vi "V_GetShapeResultNames.vi"(10 "SetParameter":T1={"Enum_ShapeType"=enum."Circles", "MaxParticle"=1, "Descriptor"={"Set 1"=100.0, "Set 2"=10.0, "Set 3"=200.0, "Set 4"=10.0}, "Match Options"={"Rotation"=TRUE, "Scale"=FALSE, "Occlusion"=FALSE, "Range Settings"=[{"Match Constraints"=0, "Min"=0.0, "Max"=360.0}]}, "Curve Parameters"={"Extraction Mode"=0, "Edge Threshold"=75, "Edge Filter Size"=1, "Min Length"=25, "Row Search Step Size"=15, "Col Search Step Size"=15, "Max Endpoint Gap"=10, "Closed"=FALSE, "Subpixel"=FALSE}, " score"=500.0} {"score" format="%#_15g"; "Curve Parameters"."Extraction Mode" items=["Normal", "Uniform Regions"]; "Curve Parameters"."Edge Filter Size" items=["Fine", "Normal"]; "Match Options"."Range Settings"."Match Constraints" items=["Rotation Angle (degrees)", "Scale Factor (%)", "Occlusion (%)"]}, 11 "ROI_Name":string="ROI1") -> (3 "ResultNames":string[](array[string]))   [LabVIEW 2019]
uses:
  Controls/Circle/Analysis_Circle_Result.ctl
  Controls/ShapeDectect/Analysis_ShapeDectect_Parameter.ctl
panel:
  in  "Tab Control":T2(tab)
  in  "Circles":T3
  in  "Ellipses":T4
  in  "Lines":T5
  in  "Rectangles":T6
  in  "Analysis_Clamp_Result":T7 {"Fitted Circle"."Average SNR (dB)" format="%.2f"; "Fitted Circle"."Average Strength" format="%.2f"; "Fitted Circle"."Roundness (Real-World)" format="%.2f"; "Fitted Circle"."Radius (Real-World)" format="%.2f"; "Fitted Circle"."Center (Real-World)"."Y" format="%.2f"; "Fitted Circle"."Center (Real-World)"."X" format="%.2f"; "Fitted Circle"."Radius (Pixels)" format="%.2f"; "Fitted Circle"."Center (Pixels)"."Y" format="%.2f"; "Fitted Circle"."Center (Pixels)"."X" format="%.2f"}
  out "error out":errorcluster
  in  "error in (no error)":errorcluster
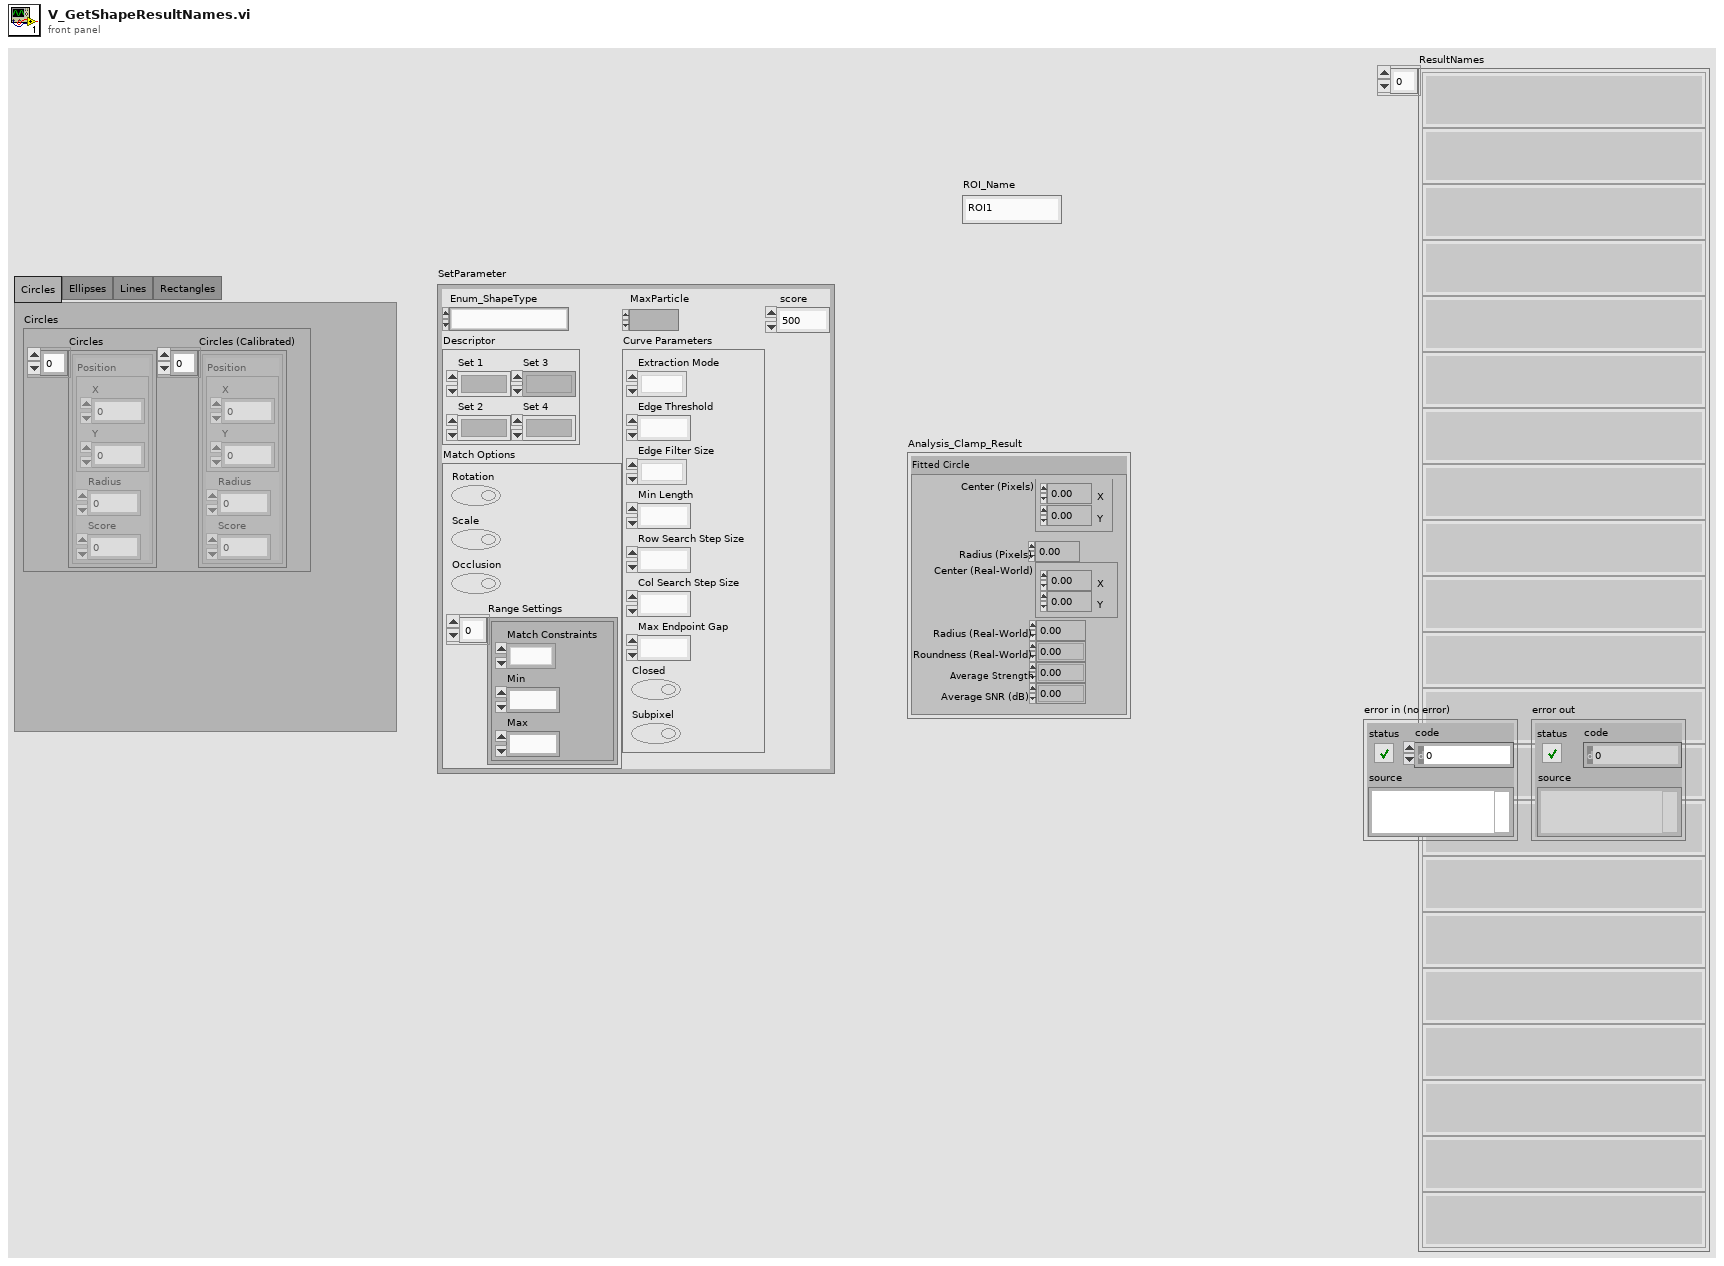
[diagram p1: front panel]
types:
  T1 = typedef "Analysis_ShapeDectect_Parameter.ctl" = cluster{"Enum_ShapeType":enum16{"Circles", "Ellipses", "Lines", "Rectangles"}, "MaxParticle":i32, "Descriptor":cluster{"Set 1":dbl, "Set 2":dbl, "Set 3":dbl, "Set 4":dbl}, "Match Options":cluster{"Rotation":bool, "Scale":bool, "Occlusion":bool, "Range Settings":cluster{"Match Constraints":u32, "Min":dbl, "Max":dbl}[]}, "Curve Parameters":cluster{"Extraction Mode":u32, "Edge Threshold":i32, "Edge Filter Size":u32, "Min Length":i32, "Row Search Step Size":i32, "Col Search Step Size":i32, "Max Endpoint Gap":i32, "Closed":bool, "Subpixel":bool}, " score":dbl}
  T2 = enum32{"Circles", "Ellipses", "Lines", "Rectangles"}
  T3 = cluster{"Circles":cluster{"Position":cluster{"X":sgl, "Y":sgl}, "Radius":dbl, "Score":dbl}[], "Circles (Calibrated)":cluster{"Position":cluster{"X":sgl, "Y":sgl}, "Radius":dbl, "Score":dbl}[]}
  T4 = cluster{"Pixel":cluster{"Position":cluster{"X":sgl, "Y":sgl}, "Angle":dbl, "Major Radius":dbl, "Minor Radius":dbl, "Score":dbl}[], "Ellipses (Calibrated)":cluster{"Position":cluster{"X":sgl, "Y":sgl}, "Orientation":dbl, "Major Radius":dbl, "Minor Radius":dbl, "Score":dbl}[]}
  T5 = cluster{"Lines":cluster{"Start Point":cluster{"X":sgl, "Y":sgl}, "End Point":cluster{"X":sgl, "Y":sgl}, "Length":dbl, "Angle":dbl, "Score":dbl}[], "Lines Calibrated":cluster{"Start Point":cluster{"X":sgl, "Y":sgl}, "End Point":cluster{"X":sgl, "Y":sgl}, "Length":dbl, "Orientation":dbl, "Score":dbl}[]}
  T6 = cluster{"Rectangles":cluster{"Corners":cluster{"X":sgl, "Y":sgl}[], "Angle":dbl, "Width":dbl, "Height":dbl, "Score":dbl}[], "Rectangles Calibrated":cluster{"Corners":cluster{"X":sgl, "Y":sgl}[], "Angle":dbl, "Width":dbl, "Height":dbl, "Score":dbl}[]}
  T7 = typedef "Analysis_Circle_Result.ctl" = cluster{"Fitted Circle":cluster{"Center (Pixels)":cluster{"X":sgl, "Y":sgl}, "Radius (Pixels)":dbl, "Center (Real-World)":cluster{"X":sgl, "Y":sgl}, "Radius (Real-World)":dbl, "Roundness (Real-World)":dbl, "Average Strength":dbl, "Average SNR (dB)":dbl}}
  T8 = enum16{"Circles", "Ellipses", "Lines", "Rectangles"}
  T9 = cluster{"Position":cluster{"X":sgl, "Y":sgl}, "Angle":dbl, "Major Radius":dbl, "Minor Radius":dbl, "Score":dbl}
  T10 = cluster{"Start Point":cluster{"X":sgl, "Y":sgl}, "End Point":cluster{"X":sgl, "Y":sgl}, "Length":dbl, "Angle":dbl, "Score":dbl}
  T11 = cluster{"Corners":cluster{"X":sgl, "Y":sgl}[], "Angle":dbl, "Width":dbl, "Height":dbl, "Score":dbl}
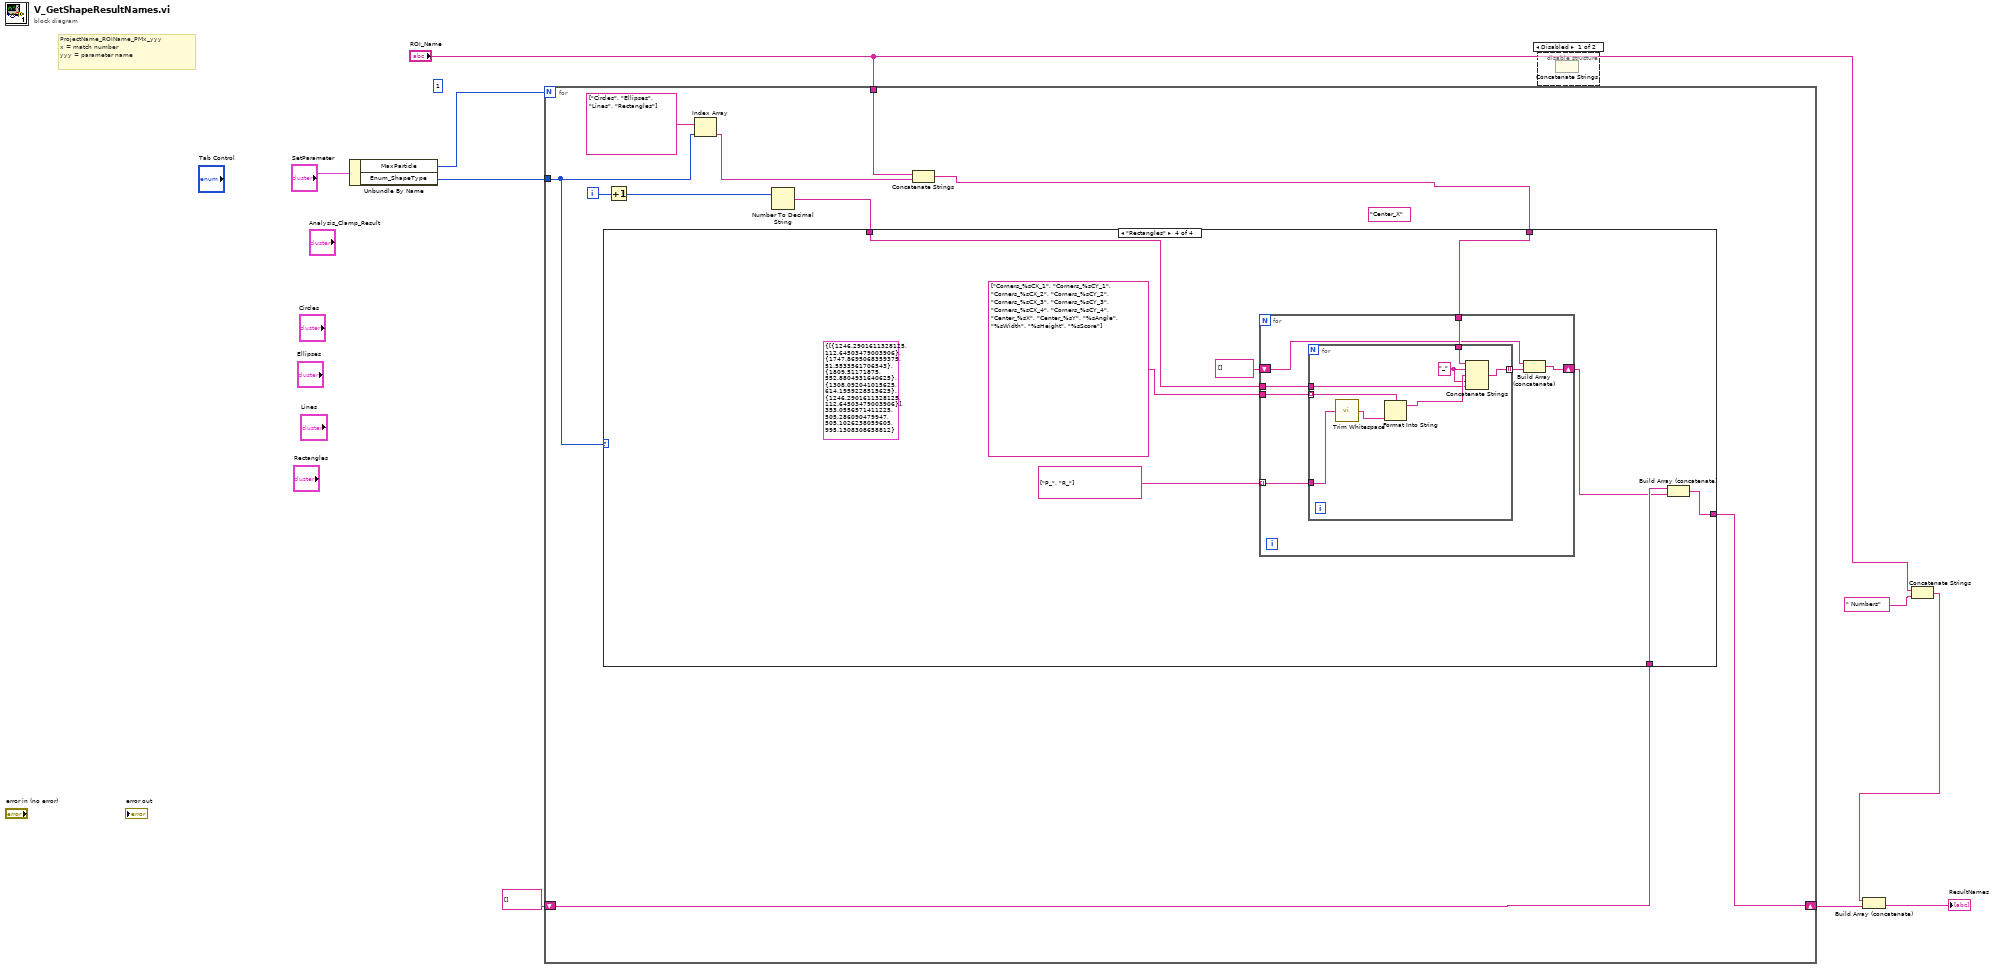
[diagram p0: block diagram]
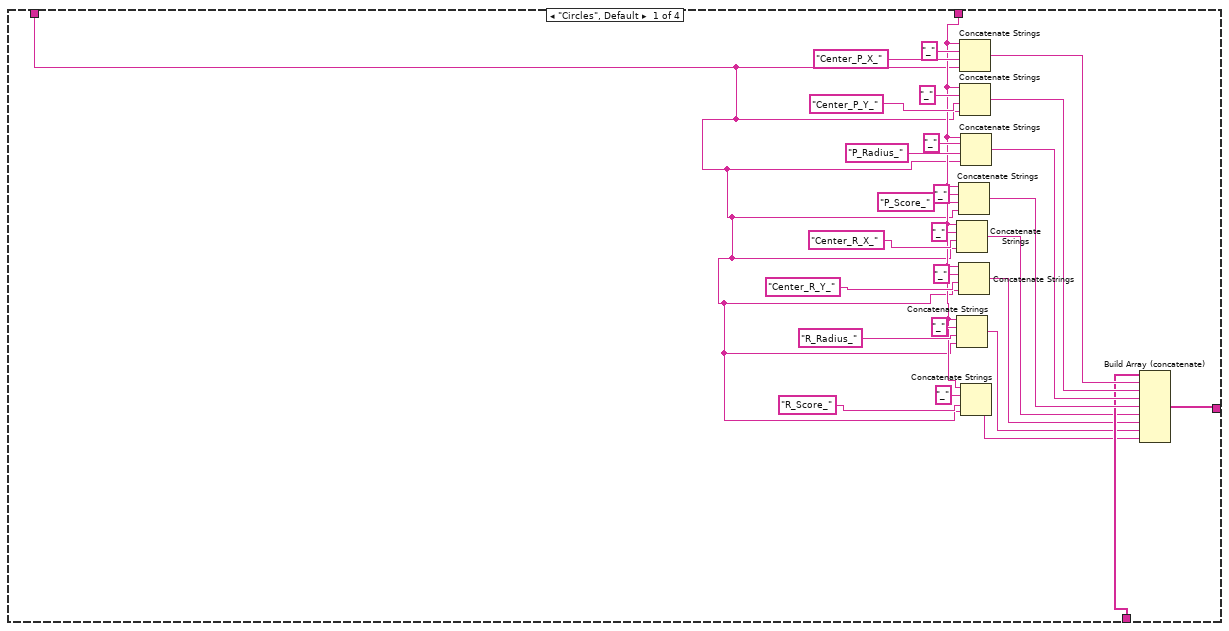
[diagram p3: hidden frame]
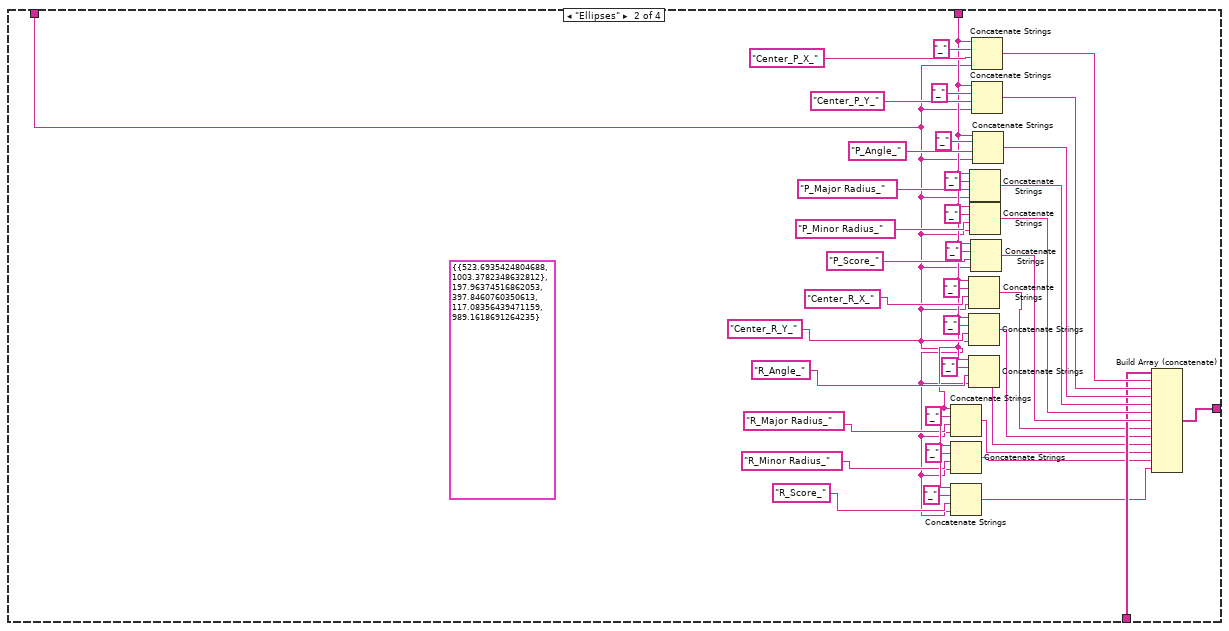
[diagram p4: hidden frame]
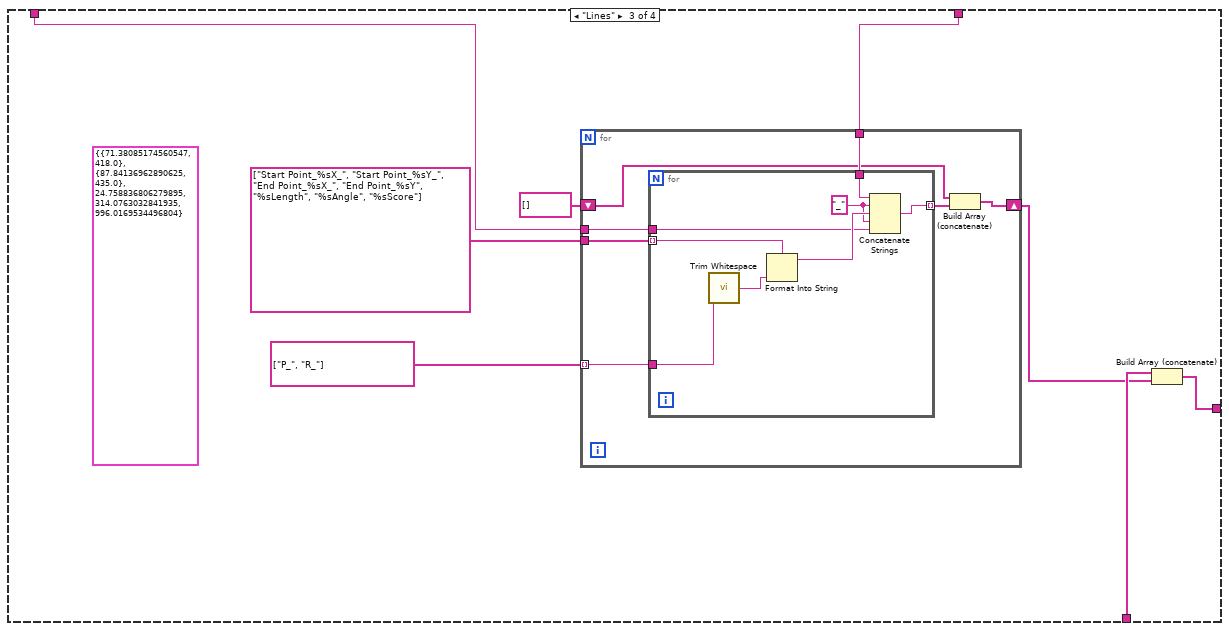
[diagram p5: hidden frame]
diagram:
  (unwired) 1 ("x")
  # "ProjectName_ROIName_PMx_yyy\nx = match number\nyyy = parameter name"
  n1 = Unbundle By Name("SetParameter") -> ("MaxParticle"=w2:i32, "Enum_ShapeType"=w6:T8)
  n2 = for {
    N: w2 -> [_]
    tunnel: "ROI_Name" -> [w18]
    shift-right: [w15] -> w8
    shift-left: string[] [] -> [w16]
    tunnel: w6 -> [w11]
    i -> [w17]
    (unwired) "Center_X" ("string")
    n3 = Increment(x=w17) -> (x+1=w19:i32)
    n4 = Index Array(array=string[] ["Circles", "Ellipses", "Lines", "Rectangles"] ("Array"), index=w11) -> (element=w12:string)
    n5 = Number To Decimal String(number=w19) -> (decimal integer string=w10:string)  [unwired: 1 in]
    n6 = Concatenate Strings(w18, w12) -> (w14:string)
    n7 = case shown="\"Rectangles\"" w11 {
      tunnel: w16 -> [w35 w55 w94 w117]
      tunnel: [w36 w87 w95 w118] -> w15
      tunnel: w14 -> [w26 w60 w91 w115]
      tunnel: w10 -> [w20 w48 w88 w111]
      frame "Circles", Default {
        n8 = Concatenate Strings(w26, "_" ("string"), "Center_R_X_" ("string"), w20) -> (w24:string)
        n9 = Concatenate Strings(w26, "_" ("string"), "R_Radius_" ("string"), w20) -> (w22:string)
        n10 = Concatenate Strings(w26, "_" ("string"), "P_Score_" ("string"), w20) -> (w45:string)
        n11 = Concatenate Strings(w26, "_" ("string"), "Center_R_Y_" ("string"), w20) -> (w23:string)
        n12 = Concatenate Strings(w26, "_" ("string"), "Center_P_X_" ("string"), w20) -> (w47:string)
        n13 = Concatenate Strings(w26, "_" ("string"), "Center_P_Y_" ("string"), w20) -> (w46:string)
        n14 = Concatenate Strings(w26, "_", "P_Radius_" ("string"), w20) -> (w37:string)
        n15 = Concatenate Strings(w26, "_" ("string"), "R_Score_" ("string"), w20) -> (w21:string)
        n16 = Build Array (concatenate)(w35, w47, w46, w37, w45, w24, w23, w22, w21) -> (w36:string[])
      }
      frame "Ellipses" {
        (unwired) T9 {"Position"={"X"=523.69354, "Y"=1003.37823}, "Angle"=197.96374516862053, "Major Radius"=397.8460760350613, "Minor Radius"=117.08356439471159, "Score"=989.1618691264235} ("Circle Descriptor")
        n17 = Concatenate Strings(w60, "_" ("string"), "R_Major Radius_" ("string"), w48) -> (w51:string)
        n18 = Concatenate Strings(w60, "_" ("string"), "R_Minor Radius_" ("string"), w48) -> (w50:string)
        n19 = Concatenate Strings(w60, "_" ("string"), "R_Score_" ("string"), w48) -> (w49:string)
        n20 = Concatenate Strings(w60, "_" ("string"), "Center_R_X_" ("string"), w48) -> (w54:string)
        n21 = Concatenate Strings(w60, "_" ("string"), "Center_R_Y_" ("string"), w48) -> (w53:string)
        n22 = Concatenate Strings(w60, "_" ("string"), "R_Angle_" ("string"), w48) -> (w52:string)
        n23 = Concatenate Strings(w60, "_" ("string"), "P_Major Radius_" ("string"), w48) -> (w84:string)
        n24 = Concatenate Strings(w60, "_" ("string"), "P_Minor Radius_" ("string"), w48) -> (w83:string)
        n25 = Concatenate Strings(w60, "_" ("string"), "P_Score_" ("string"), w48) -> (w82:string)
        n26 = Concatenate Strings(w60, "_" ("string"), "Center_P_X_" ("string"), w48) -> (w86:string)
        n27 = Concatenate Strings(w60, "_" ("string"), "Center_P_Y_" ("string"), w48) -> (w85:string)
        n28 = Concatenate Strings(w60, "_", "P_Angle_" ("string"), w48) -> (w72:string)
        n29 = Build Array (concatenate)(w55, w86, w85, w72, w84, w83, w82, w54, w53, w52, w51, w50, w49) -> (w87:string[])
      }
      frame "Lines" {
        (unwired) T10 {"Start Point"={"X"=71.38085, "Y"=418.0}, "End Point"={"X"=87.84137, "Y"=435.0}, "Length"=24.758836806279895, "Angle"=314.0763032841935, "Score"=996.0169534496804} ("Circle Descriptor")
        n30 = for {
          tunnel: string[] ["Start Point_%sX_", "Start Point_%sY_", "End Point_%sX_", "End Point_%sY", "%sLength", "%sAngle", "%sScore"] -> [w102]
          tunnel: string[] ["P_", "R_"] -> [w101] mode=indexing
          tunnel: w91 -> [w100]
          shift-right: [w98] -> w89
          shift-left: string[] [] -> [w97]
          tunnel: w88 -> [w96]
          n31 = for {
            tunnel: w102 -> [w107] mode=indexing
            tunnel: w101 -> [w110]
            tunnel: w100 -> [w109]
            tunnel: [w108] -> w99 mode=indexing
            tunnel: w96 -> [w103]
            w104 = "_" ("string")
            n32 = call <vilib>:"Trim Whitespace.vi"("string"=w110) -> ("trimmed string"=w105:string)  [unwired: 1 in]
            n33 = Format Into String(format string=w107, w105) -> (resulting string=w106:string)  [unwired: 2 in, 1 out]
            n34 = Concatenate Strings(w109, w104, w106, w104, w103) -> (w108:string)
          }
          n35 = Build Array (concatenate)(w97, w99) -> (w98:string[])
        }
        n36 = Build Array (concatenate)(w94, w89) -> (w95:string[])
      }
      frame "Rectangles" {
        (unwired) T11 {"Corners"=[{"X"=1246.2902, "Y"=112.645035}, {"X"=1747.8695, "Y"=51.553356}, {"X"=1809.5117, "Y"=552.8805}, {"X"=1308.092, "Y"=614.1959}, {"X"=1246.2902, "Y"=112.645035}], "Angle"=353.0556571411225, "Width"=505.286090479947, "Height"=505.1026238059605, "Score"=995.1308308658812} ("Rectangle Descriptor 2")
        n37 = for {
          tunnel: string[] ["Corners_%sCX_1", "Corners_%sCY_1", "Corners_%sCX_2", "Corners_%sCY_2", "Corners_%sCX_3", "Corners_%sCY_3", "Corners_%sCX_4", "Corners_%sCY_4", "Center_%sX", "Center_%sY", "%sAngle", "%sWidth", "%sHeight", "%sScore"] ("appended array") -> [w125]
          tunnel: string[] ["P_", "R_"] -> [w124] mode=indexing
          tunnel: w115 -> [w123]
          shift-right: [w121] -> w113
          shift-left: string[] [] -> [w120]
          tunnel: w111 -> [w119]
          n38 = for {
            tunnel: w125 -> [w130] mode=indexing
            tunnel: w124 -> [w133]
            tunnel: w123 -> [w132]
            tunnel: [w131] -> w122 mode=indexing
            tunnel: w119 -> [w126]
            w127 = "_" ("string")
            n39 = call <vilib>:"Trim Whitespace.vi"("string"=w133) -> ("trimmed string"=w129:string)  [unwired: 1 in]
            n40 = Format Into String(format string=w130, w129) -> (resulting string=w128:string)  [unwired: 2 in, 1 out]
            n41 = Concatenate Strings(w132, w127, w128, w127, w126) -> (w131:string)
          }
          n42 = Build Array (concatenate)(w120, w122) -> (w121:string[])
        }
        n43 = Build Array (concatenate)(w117, w113) -> (w118:string[])
      }
    }
  }
  n44 = disable-structure shown="Disabled" {
    frame Disabled {
      n45 = Concatenate Strings() -> ()  [unwired: 2 in, 1 out]
    }
    frame Enabled {
    }
  }
  n46 = Concatenate Strings("ROI_Name", " Numbers" ("string")) -> (w3:string)
  n47 = Build Array (concatenate)(w3, w8) -> (→"ResultNames":string[])
